vi "ASI_Ask_Zposition.vi"(8 "error in":errorcluster, 11 "VISA resource name":refnum<visa-resource-name>) -> (0 "error out":errorcluster, 2 "Current Z position (um)":dbl, 3 "VISA resource name out":refnum<visa-resource-name>)   [LabVIEW 2012]
panel:
  in  "Axis":u16(ring)=2 items=["X", "Y", "Z"]
  out "Serial Settings:Number of Bytes at Serial Port":u32
  out "read buffer":string
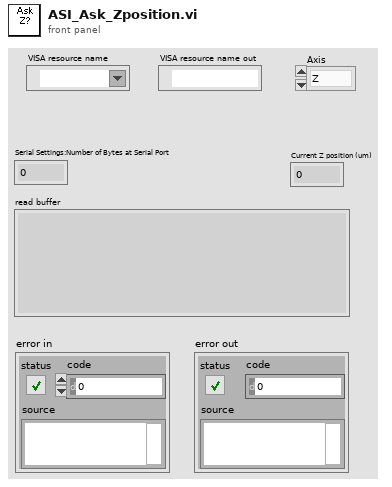
[diagram p1: front panel]
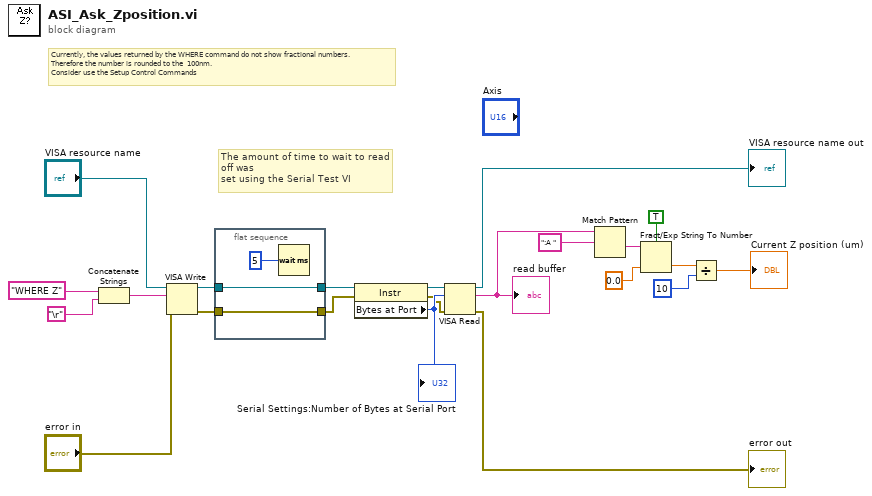
[diagram p0: block diagram]
diagram:
  # "Currently, the values returned by the WHERE command do not show fractional numbers.\nTherefore the number is rounded to the  100nm. \nConsider use the Setup Control Commands"
  # "The amount of time to wait to read off was \nset using the Serial Test VI"
  n1 = Concatenate Strings("WHERE Z" ("string"), "\r") -> (w5:string)
  n2 = VISA Write(VISA resource name="VISA resource name", write buffer=w5, error in (no error)="error in") -> (VISA resource name out=w19:refnum<visa-resource-name>, error out=w15:errorcluster)  [unwired: 1 out]
  n3 = flat-sequence {
    tunnel: [w25] -> w20
    tunnel: w19 -> [w25]
    tunnel: [w23] -> w16
    tunnel: w15 -> [w23]
    frame #0 {
      n4 = Wait (ms)(milliseconds to wait=u32 5) -> ()  [unwired: 1 out]
    }
  }
  n5 = property class="Instr"(reference=w20, error in=w16) -> (reference out=w22:refnum<visa-resource-name>, error out=w14:errorcluster, "Bytes at Port"=w21:u32)
  "Serial Settings:Number of Bytes at Serial Port" <- w21
  n6 = VISA Read(VISA resource name=w22, byte count=w21, error in (no error)=w14) -> (VISA resource name out=→"VISA resource name out":refnum<visa-resource-name>, read buffer=w11:string, error out=→"error out":errorcluster)  [unwired: 1 out]
  "read buffer" <- w11
  n7 = Match Pattern(string=w11, regular expression=":A " ("search string/char (-)")) -> (after substring=w9:string)  [unwired: 1 in, 3 out]
  n8 = Fract/Exp String To Number(use system decimal point (T)=TRUE, string=w9, default (0 dbl)=0.0 ("default (0 I32)")) -> (number=w8:dbl)  [unwired: 1 in, 1 out]
  n9 = Divide(x=w8, y=10) -> (x/y=→"Current Z position (um)":dbl)
